vi "Send LAN Event.vi"(8 "error in (no error)":errorcluster, 9 "LXI Event Edge (0: Rise)":i32(ring) items=["Rise", "Fall"], 10 "LXI Event (0: LAN0)":i32(ring) items=["LAN0", "LAN1", "LAN2", "LAN3", "LAN4", "LAN5", "LAN6", "LAN7"], 11 "VISA resource name":refnum<visa-resource-name>) -> (0 "error out":errorcluster, 3 "VISA resource name out":refnum<visa-resource-name>)   [LabVIEW 2020, in "Agilent B2900 Series.lvlib"]
doc: "Sends a LAN trigger Event."
uses:
  Agilent B2900 Series.lvlib
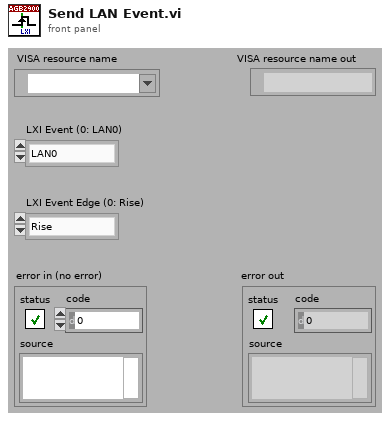
[diagram p1: front panel]
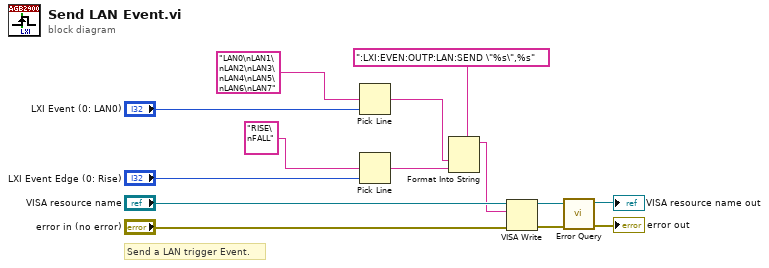
[diagram p0: block diagram]
diagram:
  # "Send a LAN trigger Event."
  n1 = Pick Line(multi-line string="LAN0\nLAN1\nLAN2\nLAN3\nLAN4\nLAN5\nLAN6\nLAN7", line index="LXI Event (0: LAN0)") -> (output string=w5:string)  [unwired: 1 in]
  n2 = Pick Line(multi-line string="RISE\nFALL", line index="LXI Event Edge (0: Rise)") -> (output string=w3:string)  [unwired: 1 in]
  n3 = Format Into String(format string=":LXI:EVEN:OUTP:LAN:SEND \"%s\",%s", w5, w3) -> (resulting string=w1:string)  [unwired: 2 in, 1 out]
  n4 = VISA Write(VISA resource name="VISA resource name", write buffer=w1, error in (no error)="error in (no error)") -> (VISA resource name out=w12:refnum<visa-resource-name>, error out=w11:errorcluster)  [unwired: 1 out]
  n5 = call "Error Query.vi"("error in (no error)"=w11, "VISA resource name"=w12) -> ("error out"=→"error out":errorcluster, "VISA resource name out"=→"VISA resource name out":refnum<visa-resource-name>)  [unwired: 6 in, 2 out]
